vi "Initialise.vi"(8 "error in (no error)":errorcluster, 11 "Node in":refnum<class "abs_Type Leaf.lvclass">) -> (0 "error out":errorcluster, 3 "Node out":refnum<class "abs_Type Leaf.lvclass">)   [LabVIEW 2021, in "BT AbsType.lvlib" / "abs_Type Leaf.lvclass"]
uses:
  abs_Type Leaf.lvclass
  abs_Type Leaf.lvclass/abs_Type Leaf.ctl
  Properties/Read Value Class.vi
  Properties/Write Value Class.vi
  <vilib>/TSA/Abstract Data Classes/Abs_Types/Type/Abs_Type.lvclass
  Source/Support/Nodes/Leaves/Leaf/bt_Leaf.lvclass
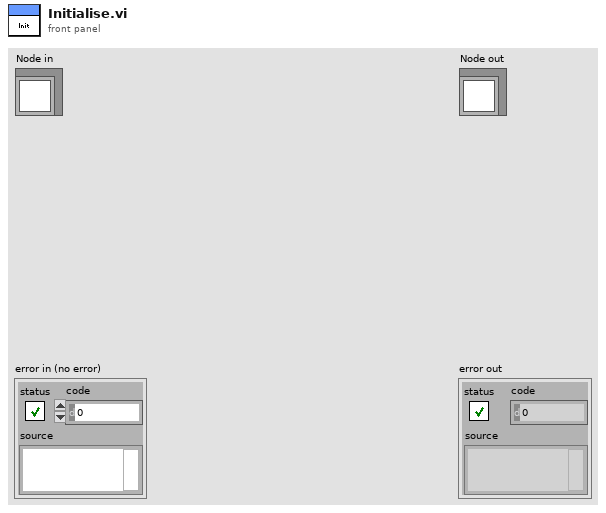
[diagram p1: front panel]
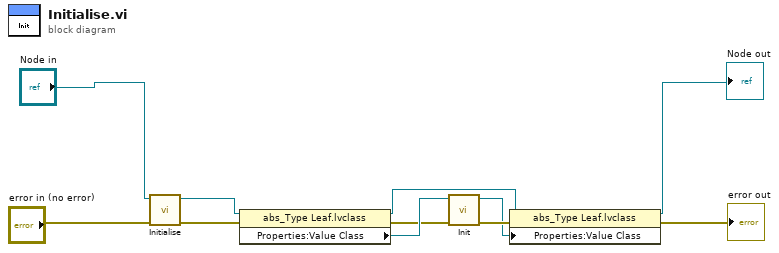
[diagram p0: block diagram]
diagram:
  n1 = call-parent "Initialise.vi"("error in (no error)"="error in (no error)", "Node in"="Node in") -> ("error out"=w7:errorcluster, "Node out"=w6:refnum<class "abs_Type Leaf.lvclass">)  [unwired: 8 in]
  n2 = property class="abs_Type Leaf.lvclass"(reference=w6, error in=w7) -> (reference out=w5:refnum<class "abs_Type Leaf.lvclass">, error out=w3:errorcluster, "Properties:Value Class"=w4:refnum<class "Abs_Type.lvclass">)
  n3 = call-dynamic "Init.vi"("error in (no error)"=w3, "Data in"=w4) -> ("error out"=w2:errorcluster, "Data out"=w1:refnum<class "Abs_Type.lvclass">)  [unwired: 8 in]
  n4 = property class="abs_Type Leaf.lvclass"(reference=w5, error in=w2, "Properties:Value Class"=w1) -> (reference out=→"Node out":refnum<class "abs_Type Leaf.lvclass">, error out=→"error out":errorcluster)
